vi "Recieve Bank Shot Result.vi"(8 "error in (no error)":errorcluster, 10 "Shot data":T1, 11 "Cap Bank Server in":refnum<class "Cap Bank Server.lvclass">) -> (0 "error out":errorcluster, 3 "Cap Bank Server out":refnum<class "Cap Bank Server.lvclass">)   [LabVIEW 2015, in "Cap Bank Server.lvclass"]
uses:
  Cap Bank Server.lvclass
  User Cap Bank/Labview/Library/Shot data.ctl
  Cap Bank Server.lvclass/Cap Bank Server.ctl
  <vilib>/ActorFramework/Actor/Actor.lvclass/Actor.ctl
  <vilib>/ActorFramework/Message Enqueuer/Message Enqueuer.lvclass/Message Enqueuer.ctl
  <vilib>/ActorFramework/Message Enqueuer/Init from Existing Queue.vi
  <vilib>/ActorFramework/Message Enqueuer/Enqueue.vi
  <vilib>/ActorFramework/Message Priority Queue/Priority Enqueue.vi
  <vilib>/ActorFramework/Message Enqueuer/Message Enqueuer.lvclass
  Mag Lab Measure Controller Messages/Log Results Msg/Log Results Msg.lvclass
  <vilib>/ActorFramework/Actor/Actor.lvclass
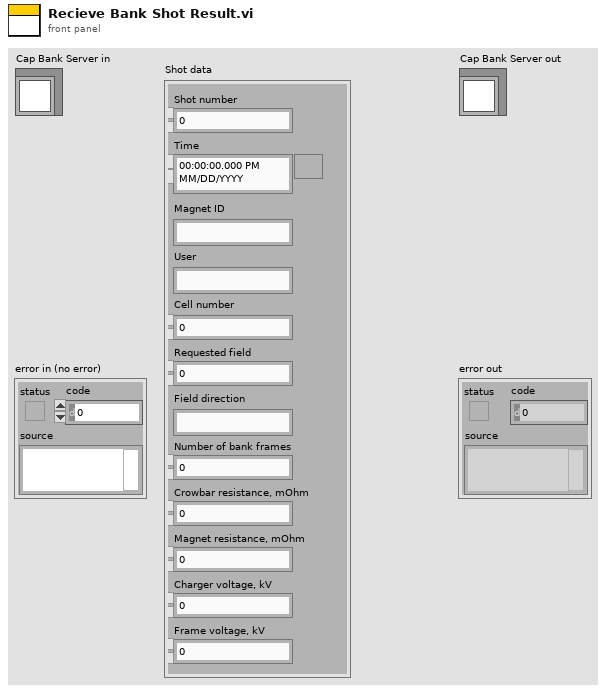
[diagram p1: front panel]
types:
  T1 = typedef "Shot data.ctl" = cluster{"Shot number":i32, "Time":timestamp, "Magnet ID":string, "User":string, "Cell number":i32, "Requested field":dbl, "Field direction":string, "Number of bank frames":i32, "Crowbar resistance, mOhm":dbl, "Magnet resistance, mOhm":dbl, "Charger voltage, kV":dbl, "Frame voltage, kV":dbl}
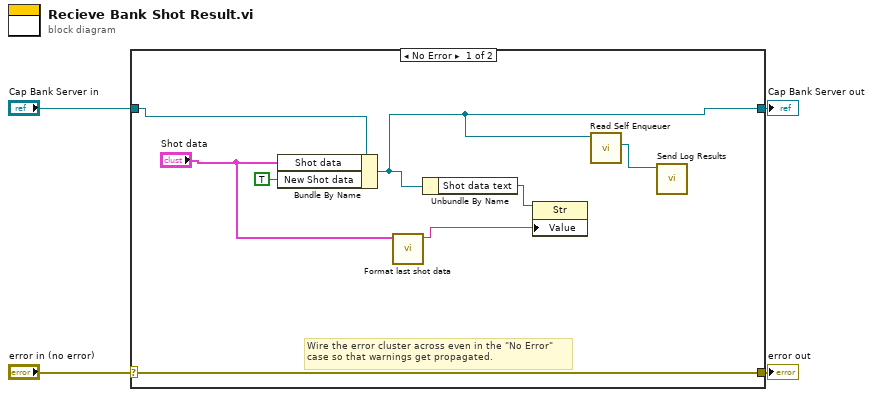
[diagram p0: block diagram]
diagram:
  n1 = case shown="No Error" "error in (no error)" {
    selector: "error in (no error)" -> [w12 w14]
    tunnel: [w12 w14] -> w3
    tunnel: [w8 w13] -> w1
    tunnel: "Cap Bank Server in" -> [w9 w13]
    frame No Error {
      # "Wire the error cluster across even in the \"No Error\"\ncase so that warnings get propagated."
      n2 = Bundle By Name(cluster=w9, "Shot data"="Shot data", "New Shot data"=TRUE ("New Idot data")) -> (w8:refnum<class "Cap Bank Server.lvclass">)
      n3 = call "Format last shot data.vi"("Shot data"="Shot data") -> ("Formated shot data"=w5:string)  [unwired: 6 in, 4 out]
      n4 = Unbundle By Name(w8) -> ("Shot data text"=w7:refnum<vi>)
      n5 = property class="Str"(reference=w7, "Value"=w5) -> ()  [unwired: 1 in, 2 out]
      n6 = call <vilib>:"Read Self Enqueuer.vi"("Actor"=w8) -> ("Self Enqueuer"=w10:refnum<class "Message Enqueuer.lvclass">)  [unwired: 10 in]
      n7 = call "Send Log Results.vi"("Message Enqueuer"=w10) -> ()  [unwired: 9 in, 2 out]
    }
    frame Error {
    }
  }
  "error out" <- w3
  "Cap Bank Server out" <- w1
